vi "Read DefaultPanelNumber.vi"(10 "error in":errorcluster caption="错误输入（无错误）") -> (2 "error out":errorcluster caption="错误输出", 3 "PanelNumber":i32 caption="值")   [LabVIEW 2016]
uses:
  <vilib>/Utility/config.llb/NI_LVConfig.lvlib
  <vilib>/Utility/config.llb/Read Key (I32).vi
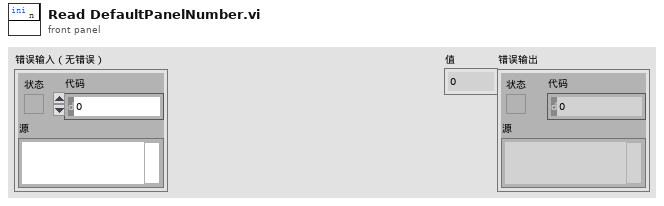
[diagram p1: front panel]
types:
  T1 = cluster{"BuildsFolder":path, "data Folder":path, "Save Folder":path, "File Folder":path, "Png Folder":path, "System ini":path, "DH Folder":path, "PageConfig":path, "DAQ Cfg Folder":path}
  T2 = typedef "NI_LVConfig.lvlib/Config Data RefNum.ctl" = refnum<k1>
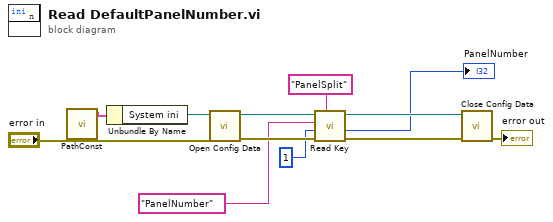
[diagram p0: block diagram]
diagram:
  n1 = call "PathConst.vi"() -> ("PathConst"=w12:T1)  [unwired: 11 in]
  n2 = Unbundle By Name(w12) -> ("System ini"=w11:path)
  n3 = call <vilib>:"Open Config Data.vi"("error in (no error)"="error in", "configuration file path"=w11) -> ("error out"=w10:errorcluster, "refnum"=w8:T2)  [unwired: 7 in, 1 out]
  n4 = call-poly <vilib>:"Read Key.vi"("section"="PanelSplit", "error in (no error)"=w10, "default value"=1, "key"="PanelNumber", "refnum"=w8) -> ("error out"=w9:errorcluster, "value"=→"PanelNumber":i32, "refnum out"=w7:T2)  [unwired: 3 in, 1 out]
  n5 = call <vilib>:"Close Config Data.vi"("error in (no error)"=w9, "refnum"=w7) -> ("error out"=→"error out":errorcluster)  [unwired: 8 in, 1 out]
